vi "Fitts_2d.vi"(11 "ID":dbl) -> (1 "W":dbl, 2 "D":dbl)   [LabVIEW 2011]
panel:
  out "ID":dbl
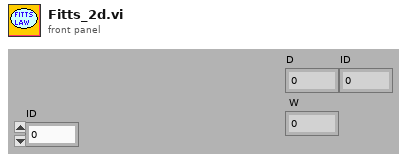
[diagram p1: front panel]
types:
  T1 = typedef "LVAllMonitorsDisplayTypeDef.ctl" = cluster{"Bounds":cluster{"Left":i16, "Top":i16, "Right":i16, "Bottom":i16}, "Depth":i16}[]
  T2 = cluster{"Bounds":cluster{"Left":i16, "Top":i16, "Right":i16, "Bottom":i16}, "Depth":i16}
  T3 = cluster{"Left":i16, "Top":i16, "Right":i16, "Bottom":i16}
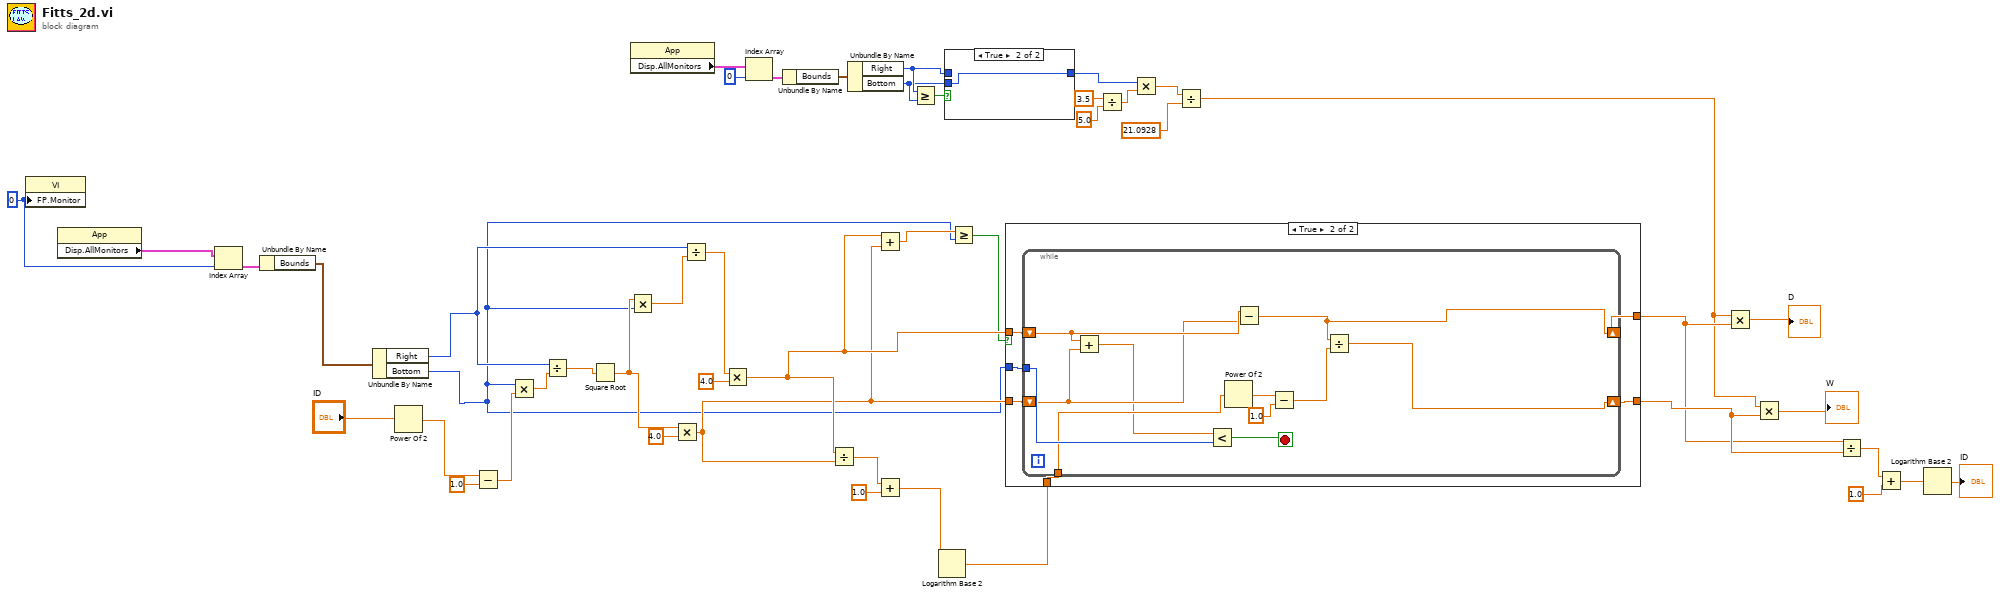
[diagram p0: block diagram]
diagram:
  w47 = u16 0 ("Front Panel Window:Monitor")
  n1 = property class="VI"("FP.Monitor"=w47) -> ()  [unwired: 2 in, 2 out]
  n2 = property class="App"() -> ("Disp.AllMonitors"=w46:T1)  [unwired: 2 in, 2 out]
  n3 = Index Array(array=w46, index=w47) -> (element=w45:T2)
  n4 = Unbundle By Name(w45) -> ("Bounds"=w44:T3)
  n5 = Unbundle By Name(w44) -> ("Right"=w9:i16, "Bottom"=w8:i16)
  n6 = Power Of 2(x="ID") -> (2^x=w41:dbl)
  n7 = Subtract(x=w41, y=1.0) -> (x-y=w39:dbl)
  n8 = Multiply(x=w8, y=w39) -> (x*y=w43:dbl)
  n9 = Divide(x=w9, y=w43) -> (x/y=w42:dbl)
  n10 = Square Root(x=w42) -> (sqrt(x)=w31:dbl)
  n11 = Multiply(x=w31, y=w8) -> (x*y=w38:dbl)
  n12 = property class="App"() -> ("Disp.AllMonitors"=w18:T1)  [unwired: 2 in, 2 out]
  n13 = Multiply(x=w31, y=4.0) -> (x*y=w27:dbl)
  n14 = Divide(x=w9, y=w38) -> (x/y=w34:dbl)
  n15 = Multiply(x=w34, y=4.0) -> (x*y=w28:dbl)
  n16 = Index Array(array=w18, index=u16 0 ("Front Panel Window:Monitor")) -> (element=w20:T2)
  n17 = Unbundle By Name(w20) -> ("Bounds"=w17:T3)
  n18 = Divide(x=w28, y=w27) -> (x/y=w37:dbl)
  n19 = Unbundle By Name(w17) -> ("Right"=w15:i16, "Bottom"=w14:i16)
  n20 = Add(x=w28, y=w27) -> (x+y=w26:dbl)
  n21 = Add(x=w37, y=1.0) -> (x+y=w35:dbl)
  n22 = Greater Or Equal?(x=w15, y=w14) -> (x >= y?=w16:bool)
  n23 = Logarithm Base 2(1:w35) -> (0:w29:dbl)
  n24 = case shown="True" w16 {
    tunnel: w15 -> [w48 _]
    tunnel: w14 -> [_ w49]
    tunnel: [w48 w49] -> w13
    frame False {
    }
    frame True {
    }
  }
  n25 = Greater Or Equal?(x=w26, y=w8) -> (x >= y?=w25:bool)
  n26 = case shown="True" w25 {
    tunnel: w29 -> [_ w57]
    tunnel: [w51 w56] -> w5
    tunnel: [w50 w55] -> w7
    tunnel: w28 -> [w51 w54]
    tunnel: w27 -> [w50 w53]
    tunnel: w8 -> [_ w52]
    frame False {
    }
    frame True {
      n27 = while {
        tunnel: w52 -> [w68]
        tunnel: w57 -> [w67]
        shift-right: [w63] -> w56
        shift-left: w54 -> [w60]
        shift-right: [w62] -> w55
        shift-left: w53 -> [w59]
        stop <- w61 stop-if-true
        n28 = Add(x=w60, y=w59) -> (x+y=w58:dbl)
        n29 = Less?(x=w58, y=w68) -> (x < y?=w61:bool)
        n30 = Power Of 2(x=w67) -> (2^x=w66:dbl)
        n31 = Subtract(x=w60, y=w59) -> (x-y=w63:dbl)
        n32 = Subtract(x=w66, y=1.0) -> (x-y=w65:dbl)
        n33 = Divide(x=w63, y=w65) -> (x/y=w62:dbl)
      }
    }
  }
  n34 = Divide(x=3.5, y=5.0) -> (x/y=w12:dbl)
  n35 = Multiply(x=w13, y=w12) -> (x*y=w10:dbl)
  n36 = Divide(x=w10, y=21.0928) -> (x/y=w3:dbl)
  n37 = Multiply(x=w3, y=w5) -> (x*y=→"D":dbl)
  n38 = Multiply(x=w3, y=w7) -> (x*y=→"W":dbl)
  n39 = Divide(x=w5, y=w7) -> (x/y=w24:dbl)
  n40 = Add(x=w24, y=1.0) -> (x+y=w22:dbl)
  n41 = Logarithm Base 2(1:w22) -> (0:→"ID":dbl)
